vi "Sensor_Reference_Sensor_v1.1_to_disassemble.vi"() -> ()   [LabVIEW 2012]
doc: "This example VI demonstrates setting up a scan list and taking a reading using the advanced VIs. For more information about the different types of VIs, see the descriptions below.\n\nEven though only two types of measurements are shown, all six types can be configured in the same way. Likewise, this VI does not show every available configurable option for voltage and resistance.\n\n====================\nSetting up and performing a scan\n====================\nThe HP34970A provides commands for setting up a scan in three ways that differ in their complexity and the amount of control offered:\n\n1. Advanced:\nEvery aspect of the measurement, scan, scan list, and read is put in a different command to allow the greatest flexibility. For example, using the advanced configure VIs, you can set up a scan list consisting of different measurement types on different channels. The \"HP34970A Advanced Scan Example.vi\" demonstrates usage of these VIs.\n\n2. Medium:\nThe instrument also offers a command that wraps up configuring individual channels and the scan list. This is represented in the driver by \"HP34970A Conf EZ.vi\". This driver specifically replaces use of the advanced configure measurement VIs and configure scan list VIs. For more information, refer to the context help for the Conf EZ VI.\n\n3. Easiest:\nThe entire configuration, scan, and read are wrapped up into one command to the instrument. This is provided in this driver as the \"EZ\" VIs, which are in the Data subpalette of the HP34970A's driver palette. The \"HP34970A EZ Scan Example.vi\" demonstrates the EZ VI's usage."
panel:
  in  "number of readings":i32=3
  out "measuring time / ms":u32
  out "measurement running":bool
  in  "current transfer ratio":dbl[unit]=1.0 caption="s"
  # "Voltage"
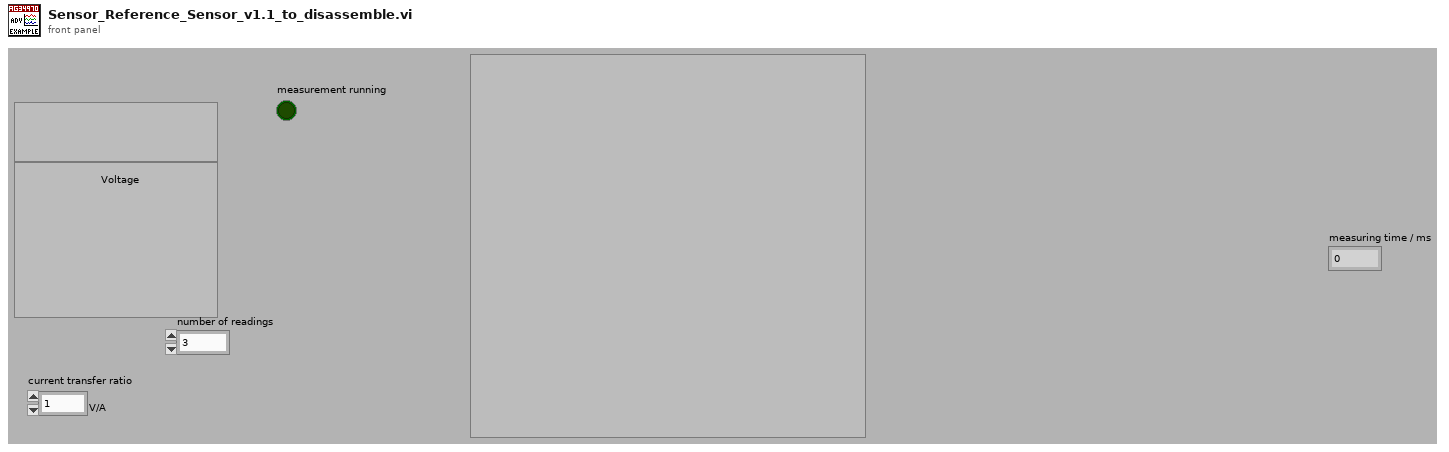
[diagram p1: front panel]
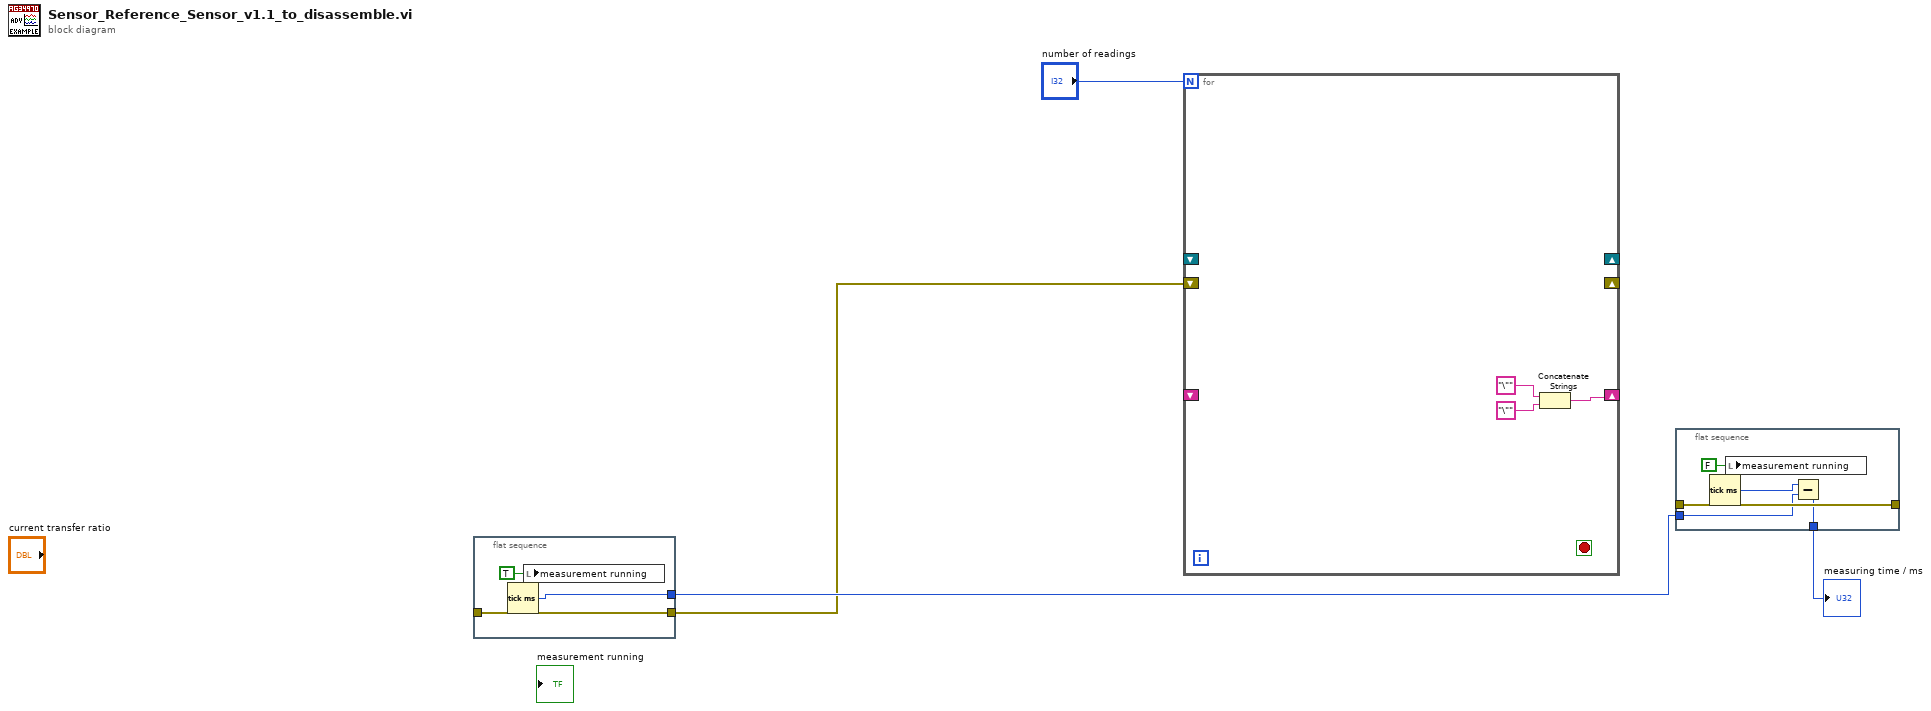
[diagram p0: block diagram]
diagram:
  n1 = flat-sequence {
    tunnel: [w9] -> w3
    tunnel: [w9] -> _
    tunnel: [w8] -> w6
    frame #0 {
      n2 = Tick Count (ms)() -> (millisecond timer value=w8:u32)
      n3 = local write "measurement running"(TRUE ("measurement running")) -> ()
    }
  }
  n4 = for {
    N: "number of readings" -> [_]
    shift-right: _ -> [_]
    shift-left: [_] -> w4
    shift-right: _ -> [_]
    shift-left: w3 -> [_]
    shift-right: [w11] -> w7
    shift-left: _ -> [_]
    stop <- w14 stop-if-true
    n5 = Concatenate Strings("\"" ("string"), "\"" ("string")) -> (w11:string)
  }
  n6 = flat-sequence {
    tunnel: [w18] -> w1
    tunnel: [w18] -> _
    tunnel: w6 -> [w16]
    tunnel: [w15] -> w5
    frame #0 {
      n7 = Tick Count (ms)() -> (millisecond timer value=w17:u32)
      n8 = local write "measurement running"(FALSE ("measurement running")) -> ()
      n9 = Subtract(x=w17, y=w16) -> (x-y=w15:u32)
    }
  }
  "measuring time / ms" <- w5
